vi "Globals.vi"() -> ()   [LabVIEW 2017, in "nifxpmath_Multiplier.xnode"]
uses:
  <vilib>/rvi/FXPMathLib/FxpMul/XNode/nifxpmath_Multiplier.xnode
panel:
  out "SMALL ICON w/ 4WIRE":picture
  out "SMALL ICON":picture
  out "NORMAL BANNER":picture
  in  "TERM X*Y NAME":string="x*y"
  in  "TERM Y NAME":string="y"
  in  "TERM X NAME":string="x"
  in  "TERM OVFL ID":string="TERM_OVFL"
  in  "TERM X*Y ID":string="TERM_XY"
  in  "TERM Y ID":string="TERM_Y"
  in  "TERM X ID":string="TERM_X"
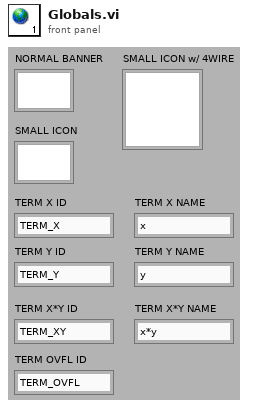
[diagram p1: front panel]
diagram:
